vi "Do.vi"(6 "Cmd":T1, 8 "error in (no error)":errorcluster, 11 "NeedleValve in":refnum<class "NeedleValve.lvclass">) -> (0 "error out":errorcluster, 3 "NeedleValve out":refnum<class "NeedleValve.lvclass">)   [LabVIEW 2019, in "NeedleValve.lvclass"]
uses:
  NeedleValve.lvclass
  D:/GIT H4000/H4000/src/Device_class/Device.lvclass
  Cmd.ctl
  Device_class/Device.lvclass/Device.ctl
  MessageInterface_class/MessageInterface.lvclass
  Device_class/Device.lvclass
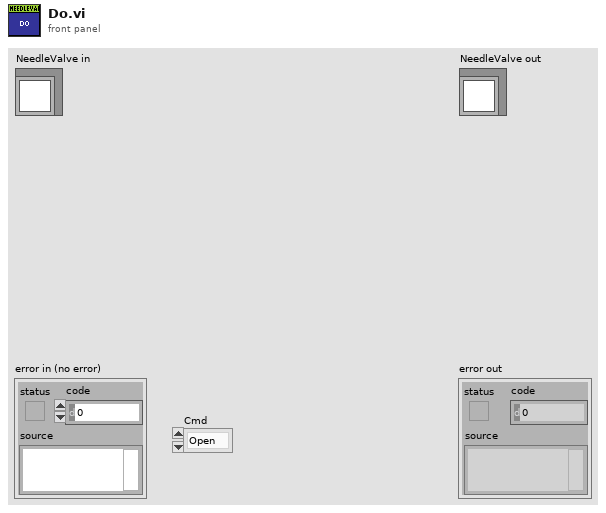
[diagram p1: front panel]
types:
  T1 = typedef "NeedleValve.lvclass/Cmd.ctl" = enum16{"Open", "Close", "Stop"}
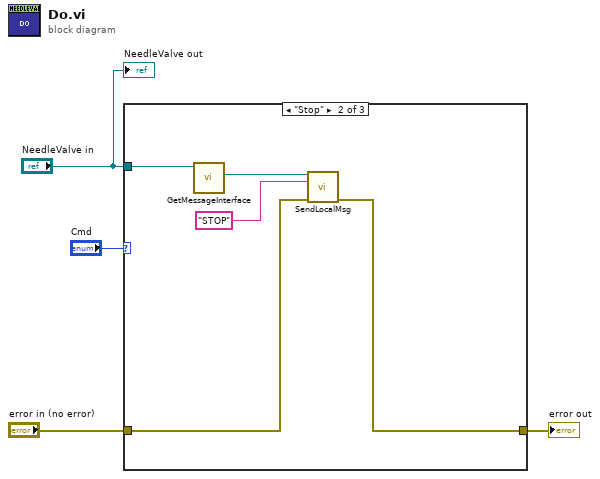
[diagram p0: block diagram]
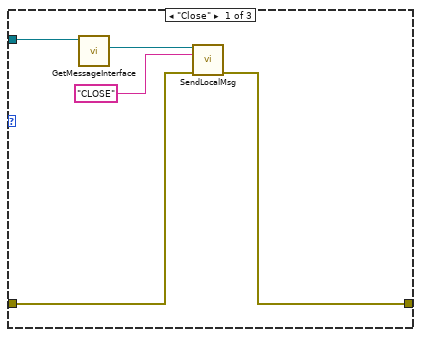
[diagram p2: hidden frame]
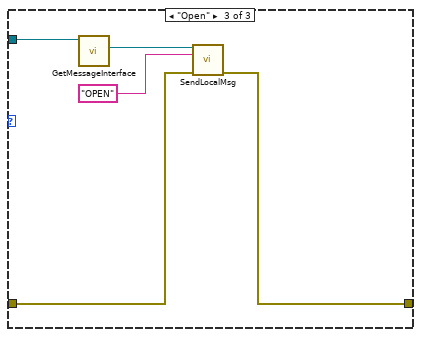
[diagram p3: hidden frame]
diagram:
  n1 = case shown="\"Stop\"" "Cmd" {
    tunnel: "error in (no error)" -> [w9 w14 w19]
    tunnel: [w8 w13 w18] -> w3
    tunnel: "NeedleValve in" -> [w7 w12 w17]
    frame "Close" {
      n2 = call "GetMessageInterface.vi"("Device in"=w7) -> ("MessageInterface"=w6:refnum<class "MessageInterface.lvclass">)  [unwired: 10 in]
      n3 = call-dynamic "SendLocalMsg.vi"("reference in"=w6, "name"="CLOSE", "error in (no error)"=w9) -> ("error out"=w8:errorcluster)  [unwired: 10 in, 2 out]
    }
    frame "Stop" {
      n4 = call "GetMessageInterface.vi"("Device in"=w12) -> ("MessageInterface"=w11:refnum<class "MessageInterface.lvclass">)  [unwired: 10 in]
      n5 = call-dynamic "SendLocalMsg.vi"("reference in"=w11, "name"="STOP", "error in (no error)"=w14) -> ("error out"=w13:errorcluster)  [unwired: 10 in, 2 out]
    }
    frame "Open" {
      n6 = call "GetMessageInterface.vi"("Device in"=w17) -> ("MessageInterface"=w16:refnum<class "MessageInterface.lvclass">)  [unwired: 10 in]
      n7 = call-dynamic "SendLocalMsg.vi"("reference in"=w16, "name"="OPEN", "error in (no error)"=w19) -> ("error out"=w18:errorcluster)  [unwired: 10 in, 2 out]
    }
  }
  "error out" <- w3
  "NeedleValve out" <- "NeedleValve in"
